vi "exp4.vi"() -> ()   [LabVIEW 2014]
uses:
  <vilib>/Instr/_visa.llb/VISA Configure Serial Port (Instr).vi
panel:
  in  "?":dbl
  in  "port":refnum<visa-resource-name>
  in  "停止":bool
  out "read string":string
  in  "string to write":string
  out "波形チャート":dbl(graph)
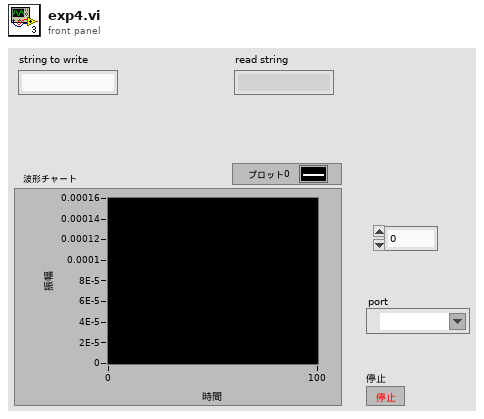
[diagram p1: front panel]
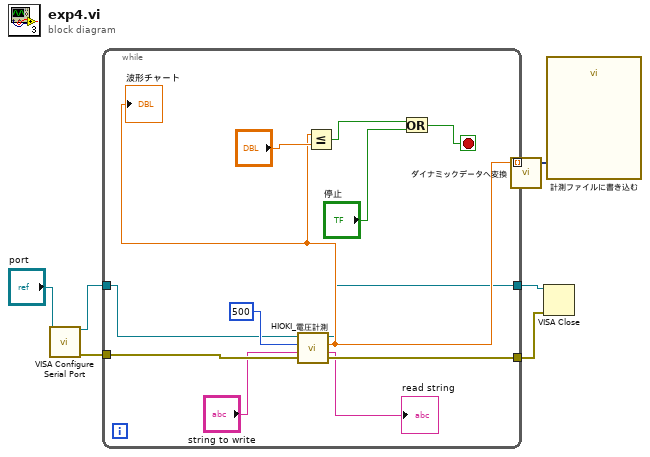
[diagram p0: block diagram]
diagram:
  n1 = call-poly "VISA Configure Serial Port"("VISA resource name"="port") -> ("VISA resource name out"=w3:refnum<visa-resource-name>, "error out"=w6:errorcluster)  [unwired: 13 in]
  n2 = while {
    tunnel: [w18] -> w7
    tunnel: w6 -> [w18]
    tunnel: [w8] -> w4
    tunnel: w3 -> [w9]
    tunnel: [w14] -> w2 mode=indexing
    stop <- w12 stop-if-true
    n3 = call "HIOKI_電圧計測.vi"("VISA resource name out 2"=w9, "delay before read (ms)"=500, "string to write"="string to write") -> ("VISA resource name out"=w8:refnum<visa-resource-name>, "数値"=w14:dbl, "read string"=→"read string":string)  [unwired: 1 in, 2 out]
    "波形チャート" <- w14
    n4 = Less Or Equal?(x=w14, y="?") -> (x <= y?=w13:bool)
    n5 = Or(x=w13, y="停止") -> (x .or. y?=w12:bool)
  }
  n6 = call "ダイナミックデータへ変換"("Array"=w2) -> ("Dynamic Data Type"=w1:dynamicdata)  [unwired: 3 in]
  n7 = VISA Close(VISA resource name=w4, error in (no error)=w7) -> ()  [unwired: 1 out]
  n8 = call "計測ファイルに書き込む"("Signals"=w1) -> ()  [unwired: 16 in, 3 out]
